vi "SubVI Tester.vi"() -> ()   [LabVIEW 2012]
doc: "In this challenge exercise, you add wind information to the weather data type definition."
uses:
  Weather Data.ctl
panel:
  out "Weather Data Out":T1={"Current Temperature"=0.0, "Max Temperature"=0.0, "Min Temperature"=0.0, "Temperature Warning?"=FALSE, "Temperature Warning Text"="No Warning", "Current Windspeed"=0.0, "Max Windspeed"=0.0, "Windspeed Warning?"=FALSE, "Windspeed Warning Text"="No Warning"}
  in  "Max Windspeed":dbl
  in  "Current Windspeed":dbl
  in  "Min Temperature":dbl
  in  "Max Temperature":dbl
  in  "Stop":bool
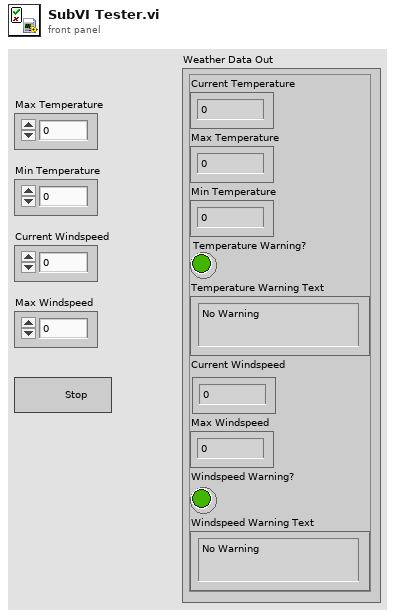
[diagram p1: front panel]
types:
  T1 = typedef "Weather Data.ctl" = cluster{"Current Temperature":dbl, "Max Temperature":dbl, "Min Temperature":dbl, "Temperature Warning?":bool, "Temperature Warning Text":string, "Current Windspeed":dbl, "Max Windspeed":dbl, "Windspeed Warning?":bool, "Windspeed Warning Text":string}
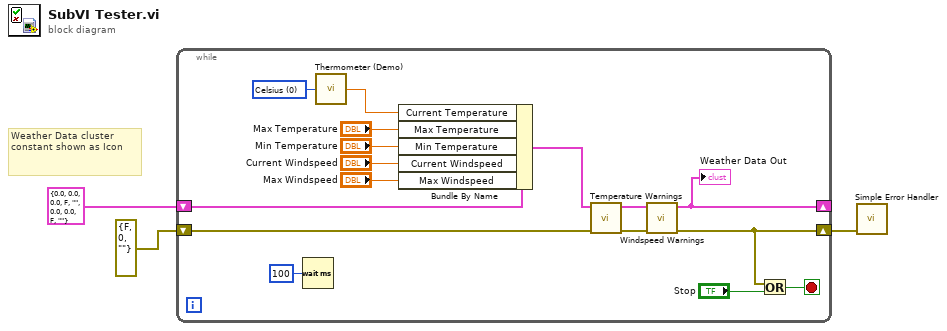
[diagram p0: block diagram]
diagram:
  # "Weather Data cluster constant shown as Icon"
  n1 = while {
    shift-right: [w12] -> _
    shift-left: T1 {"Current Temperature"=0.0, "Max Temperature"=0.0, "Min Temperature"=0.0, "Temperature Warning?"=FALSE, "Temperature Warning Text"="", "Current Windspeed"=0.0, "Max Windspeed"=0.0, "Windspeed Warning?"=FALSE, "Windspeed Warning Text"=""} ("Weather Data In") -> [w19]
    shift-right: [w13] -> w2
    shift-left: errorcluster {"status"=FALSE, "code"=0, "source"=""} ("error out") -> [w15]
    stop <- w16 stop-if-true
    w9 = u16 0 items=["Celsius", "Fahrenheit"] ("Units (0: Celsius)")
    n2 = Wait (ms)(milliseconds to wait=u32 100) -> ()  [unwired: 1 out]
    n3 = call "Thermometer (Demo).vi"("Units (0: Celsius)"=w9) -> ("Temperature Value"=w4:dbl)
    n4 = Bundle By Name(cluster=w19, "Current Temperature"=w4, "Max Temperature"="Max Temperature", "Min Temperature"="Min Temperature", "Current Windspeed"="Current Windspeed", "Max Windspeed"="Max Windspeed") -> (w11:T1)
    n5 = call "Temperature Warnings.vi"("Error In"=w15, "Weather Data In"=w11) -> ("Error Out"=w14:errorcluster, "Weather Data Out"=w10:T1)  [unwired: 8 in]
    n6 = call "Windspeed Warnings.vi"("error in"=w14, "Weather Data In"=w10) -> ("error out"=w13:errorcluster, "Weather Data Out"=w12:T1)  [unwired: 8 in]
    "Weather Data Out" <- w12
    n7 = Or(x=w13, y="Stop") -> (x .or. y?=w16:bool)
  }
  n8 = call <vilib>:"Simple Error Handler.vi"("error in (no error)"=w2) -> ()  [unwired: 4 in, 5 out]
